vi "Format Report Data(SubVI).vi"(8 "Error In":errorcluster, 10 "AE-Groups SR Data":T1[](array[typedef]), 11 "AE Group Names":string[](array[string])=["AE-Poland", "AE-Czech", "AE-Hungary", "AE-Romania"]) -> (0 "Error Out":errorcluster, 1 "SR Data Out":dbl[][](array[numeric]), 2 "Row headers":string[](array[string]), 3 "Formated SR Data Out":string[][](array[string]))   [LabVIEW 2018, in "DS_Lib.lvlib" / "SRReportParser.lvlib"]
uses:
  SRReportParser.lvlib
  TypeDefs/Weekly_SR_Stats.ctl
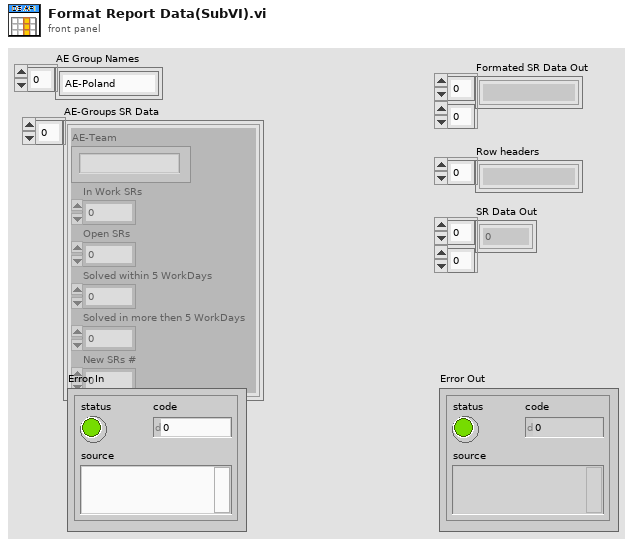
[diagram p1: front panel]
types:
  T1 = typedef "DS_Lib.lvlib/SRReportParser.lvlib/Weekly_SR_Stats.ctl" = cluster{"AE-Team":string, "In Work SRs":i32, "Open SRs":i32, "Solved within 5 WorkDays":i32, "Solved in more then 5 WorkDays":i32, "New SRs #":i32}
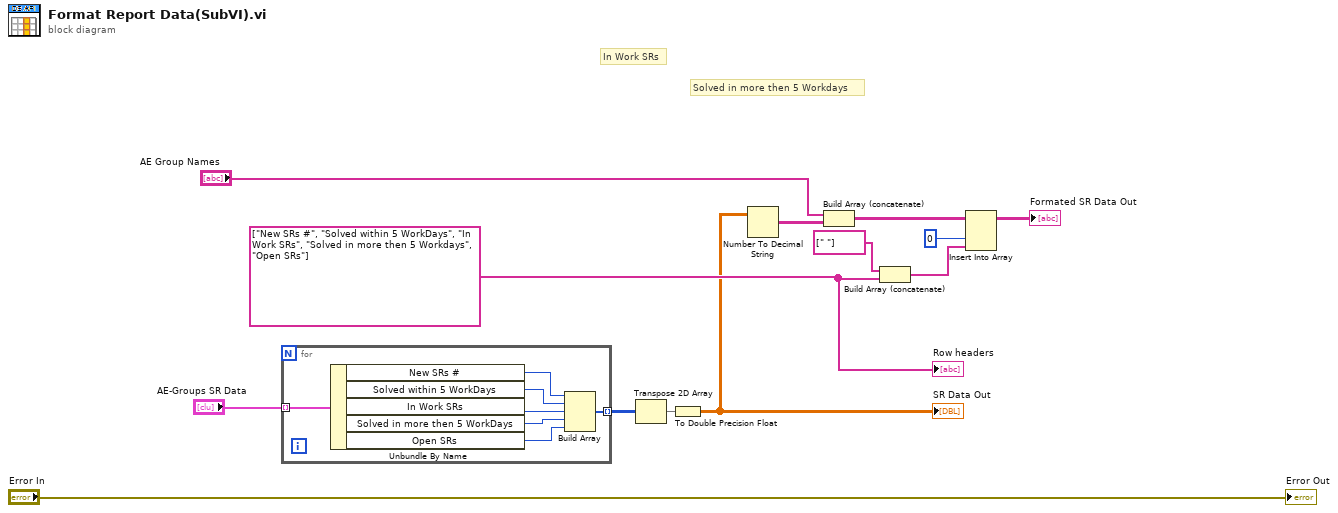
[diagram p0: block diagram]
diagram:
  w8 = string[] ["New SRs #", "Solved within 5 WorkDays", "In Work SRs", "Solved in more then 5 Workdays", "Open SRs"] ("row headers")
  # "Solved in more then 5 Workdays"
  # "In Work SRs"
  n1 = for {
    tunnel: "AE-Groups SR Data" -> [w14] mode=indexing
    tunnel: [w16] -> w3 mode=indexing
    n2 = Unbundle By Name(w14) -> ("New SRs #"=w15:i32, "Solved within 5 WorkDays"=w20:i32, "In Work SRs"=w19:i32, "Solved in more then 5 WorkDays"=w18:i32, "Open SRs"=w17:i32)
    n3 = Build Array(w15, w20, w19, w18, w17) -> (w16:i32[])
  }
  n4 = Transpose 2D Array(2D array=w3) -> (transposed array=w12:i32[][])
  n5 = To Double Precision Float(number=w12) -> (double precision float=w4:dbl[][])
  "SR Data Out" <- w4
  n6 = Number To Decimal String(number=w4) -> (decimal integer string=w5:string[][])  [unwired: 1 in]
  n7 = Build Array (concatenate)("AE Group Names", w5) -> (w6:string[][])
  n8 = Build Array (concatenate)(string[] [" "] ("element"), w8) -> (w10:string[])
  n9 = Insert Into Array(array=w6, index (col)=0 ("disabled index (col)"), new element=w10) -> (→"Formated SR Data Out":string[][])  [unwired: 1 in]
  "Row headers" <- w8
  "Error Out" <- "Error In"
